vi "row1.vi"(2 "Array in":i32[](array[numeric])) -> (0 "Array out":i32[](array[numeric]), 1 "Enum":T1(ring))   [LabVIEW 2016]
uses:
  <vilib>/NXT/Block Support/NXT_OutputPort.ctl
  <vilib>/NXT/Block Support/NXT_InputPort.ctl
  <vilib>/NXT/Subs/ColorSensorColors.ctl
  <vilib>/NXT/NXTIO Xnodes/NXTIONodeSubVIs/NXTStopMotors.vi
  <vilib>/NXT/NXTIO Xnodes/NXTIONodeSubVIs/NXTMotorRunDistance.vi
  <vilib>/NXT/NXTIO Xnodes/NXTIONodeSubVIs/LEGOMotorStatus.vi
  <vilib>/NXT/NXTIO Xnodes/NXTIONodeSubVIs/NXTMoveMotors.vi
  <vilib>/NXT/NXTIO Xnodes/NXTIONodeSubVIs/LEGOResetMotors.vi
  <vilib>/NXT/Subs/LVHSConnector.ctl
  <vilib>/NXT/NXTIO Xnodes/AddressXNode/NXTIOAddress.xnode
  <vilib>/NXT/NXTIO Xnodes/NXTIOXNode/NXTIO.xnode
  <vilib>/NXT/LegoClasses/BrickReference/BrickReference.lvclass
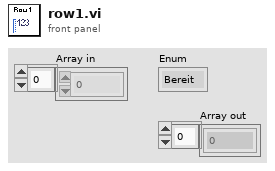
[diagram p1: front panel]
types:
  T1 = enum16{"Bereit", "Move 1", "Reference_pos", "Wait", "row1_check", "row2_check", "row3_check", "return", "move2", "move3", "move4", "move5", "end"}
  T2 = enum16{"forward", "pause1", "right1", "pause2", "right2", "pause3", "end"}
  T3 = typedef "NXT_OutputPort.ctl" = u8
  T4 = typedef "ColorSensorColors.ctl" = enum16{"No Color", "Black", "Blue", "Green", "Yellow", "Red", "White", "Brown"}
  T5 = cluster{"Output Port":T3, "Output Port 2":T3, "Output Port 3":T3}
  T6 = typedef "LVHSConnector.ctl" = refnum<class "BrickReference.lvclass">
  T7 = typedef "NXT_InputPort.ctl" = u32
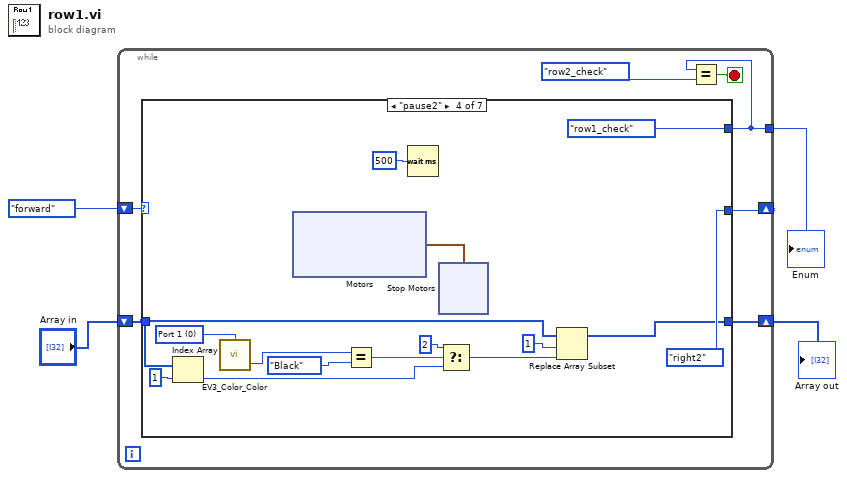
[diagram p0: block diagram]
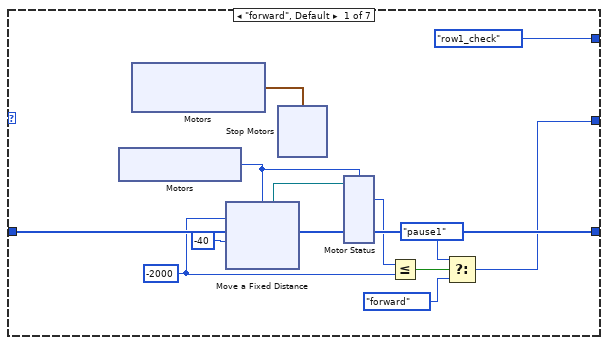
[diagram p2: hidden frame]
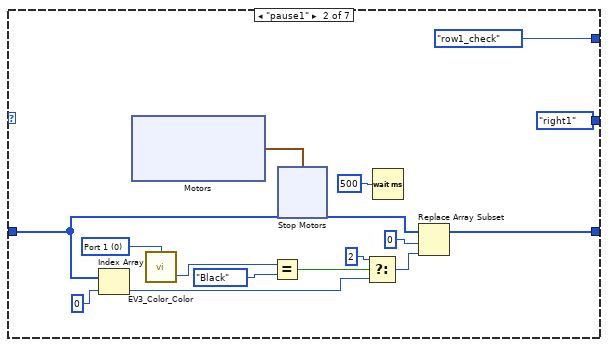
[diagram p3: hidden frame]
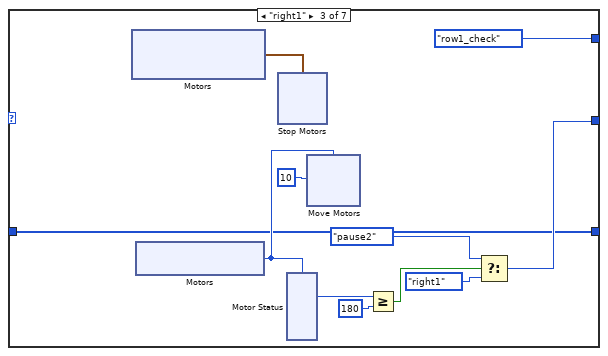
[diagram p4: hidden frame]
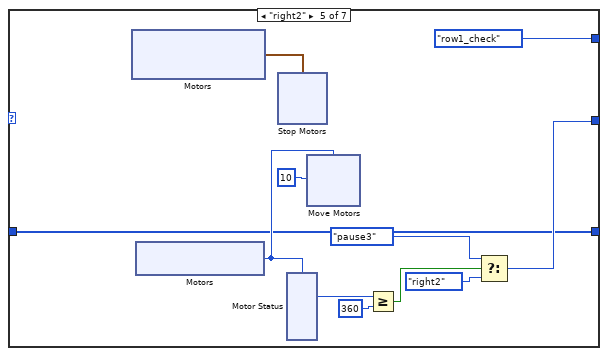
[diagram p5: hidden frame]
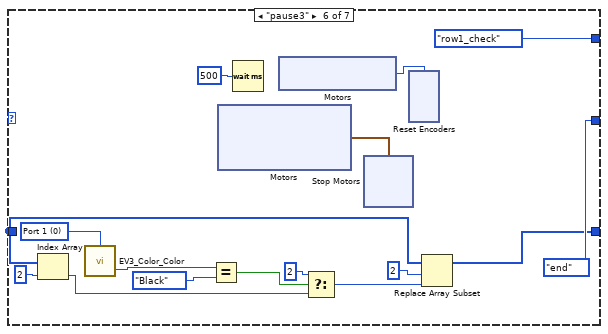
[diagram p6: hidden frame]
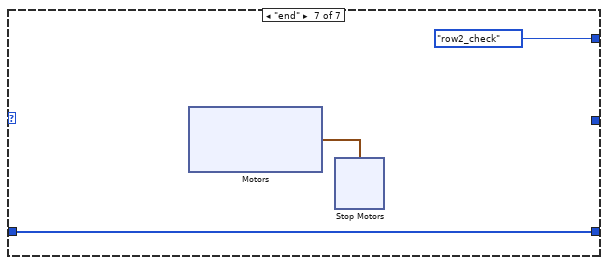
[diagram p7: hidden frame]
diagram:
  n1 = while {
    shift-right: [w10] -> _
    shift-left: T2."forward" -> [w11]
    tunnel: [w9] -> w2
    shift-right: [w7] -> w3
    shift-left: "Array in" -> [w8]
    stop <- w5 stop-if-true
    n2 = case shown="\"pause2\"" w11 {
      tunnel: [w15 T2."right1" w73 T2."right2" w129 T2."end" _] -> w10
      tunnel: [T1."row1_check" T1."row1_check" T1."row1_check" T1."row1_check" T1."row1_check" T1."row1_check" T1."row2_check"] -> w9
      tunnel: [w21 w49 w71 w105 w125 w158 w185] -> w7
      tunnel: w8 -> [w21 w51 w71 w106 w125 w159 w185]
      frame "forward", Default {
        w18 = -2000 ("Distance 1")
        n3 = xnode "Motors"() -> ("Motor"=w17:T3)
        n4 = xnode "Motors"() -> ("Motor"=w23:cluster{"Port":T3, "Port":T3})
        n5 = xnode "Move a Fixed Distance"("Speed 1"=i8 -40, "Distance 1"=w18, "Motors"=w17) -> ("NXT/EV3"=w16:T6)  [unwired: 1 in]
        n6 = xnode "Stop Motors"("Motors"=w23) -> ()  [unwired: 1 in, 1 out]
        n7 = xnode "Motor Status"("Motors"=w17, "NXT/EV3"=w16) -> ("Position 1"=w19:i32)  [unwired: 2 out]
        n8 = Less Or Equal?(x=w19, y=w18) -> (x <= y?=w12:bool)
        n9 = Select(t=T2."pause1", s=w12, f=T2."forward") -> (s? t:f=w15:T2)
      }
      frame "pause1" {
        w62 = T7 0 items=["Port 1", "Port 2", "Port 3", "Port 4"] ("Port (Port 1)")
        n10 = Index Array(array=w51, index=0 ("disabled index (col)")) -> (element=w50:i32)
        n11 = xnode "Motors"() -> ("Motor"=w63:cluster{"Port":T3, "Port":T3, "Port":T3})
        n12 = call <vilib>:"EV3_Color_Color.vi"("Port (Port 1)"=w62) -> ("Detected Color"=w61:T4)  [unwired: 2 in, 1 out]
        n13 = Equal?(x=w61, y=ColorSensorColors."Black") -> (x = y?=w58:bool)
        n14 = xnode "Stop Motors"("Motors"=w63) -> ()  [unwired: 1 in, 1 out]
        n15 = Select(t=2 ("disabled index (col)"), s=w58, f=w50) -> (s? t:f=w54:i32)
        n16 = Wait (ms)(milliseconds to wait=u32 500) -> ()  [unwired: 1 out]
        n17 = Replace Array Subset(array=w51, new element=w54, index=0 ("index (row)")) -> (w49:i32[])
      }
      frame "right1" {
        n18 = xnode "Motors"() -> ("Motor"=w78:cluster{"Port":T3, "Port":T3})
        n19 = xnode "Motors"() -> ("Motor"=w79:T3)
        n20 = xnode "Stop Motors"("Motors"=w78) -> ()  [unwired: 1 in, 1 out]
        n21 = xnode "Motor Status"("Motors"=w79) -> ("Position 1"=w77:i32)  [unwired: 1 in, 2 out]
        n22 = xnode "Move Motors"("Power/Speed 1"=i8 10, "Motors"=w79) -> ()  [unwired: 1 in, 1 out]
        n23 = Greater Or Equal?(x=w77, y=180) -> (x >= y?=w75:bool)
        n24 = Select(t=T2."pause2", s=w75, f=T2."right1") -> (s? t:f=w73:T2)
      }
      frame "pause2" {
        w116 = T7 0 items=["Port 1", "Port 2", "Port 3", "Port 4"] ("Port (Port 1)")
        n25 = Index Array(array=w106, index=1 ("disabled index (col)")) -> (element=w107:i32)
        n26 = call <vilib>:"EV3_Color_Color.vi"("Port (Port 1)"=w116) -> ("Detected Color"=w115:T4)  [unwired: 2 in, 1 out]
        n27 = xnode "Motors"() -> ("Motor"=w117:cluster{"Port":T3, "Port":T3, "Port":T3})
        n28 = Equal?(x=w115, y=ColorSensorColors."Black") -> (x = y?=w112:bool)
        n29 = Wait (ms)(milliseconds to wait=u32 500) -> ()  [unwired: 1 out]
        n30 = xnode "Stop Motors"("Motors"=w117) -> ()  [unwired: 1 in, 1 out]
        n31 = Select(t=2 ("disabled index (col)"), s=w112, f=w107) -> (s? t:f=w103:i32)
        n32 = Replace Array Subset(array=w106, new element=w103, index=1 ("disabled index (col)")) -> (w105:i32[])
      }
      frame "right2" {
        n33 = xnode "Motors"() -> ("Motor"=w132:cluster{"Port":T3, "Port":T3})
        n34 = xnode "Motors"() -> ("Motor"=w133:T3)
        n35 = xnode "Stop Motors"("Motors"=w132) -> ()  [unwired: 1 in, 1 out]
        n36 = xnode "Motor Status"("Motors"=w133) -> ("Position 1"=w128:i32)  [unwired: 1 in, 2 out]
        n37 = xnode "Move Motors"("Power/Speed 1"=i8 10, "Motors"=w133) -> ()  [unwired: 1 in, 1 out]
        n38 = Greater Or Equal?(x=w128, y=360) -> (x >= y?=w131:bool)
        n39 = Select(t=T2."pause3", s=w131, f=T2."right2") -> (s? t:f=w129:T2)
      }
      frame "pause3" {
        w171 = T7 0 items=["Port 1", "Port 2", "Port 3", "Port 4"] ("Port (Port 1)")
        n40 = Index Array(array=w159, index=2 ("disabled index (col)")) -> (element=w162:i32)
        n41 = call <vilib>:"EV3_Color_Color.vi"("Port (Port 1)"=w171) -> ("Detected Color"=w170:T4)  [unwired: 2 in, 1 out]
        n42 = Equal?(x=w170, y=ColorSensorColors."Black") -> (x = y?=w167:bool)
        n43 = xnode "Motors"() -> ("Motor"=w172:cluster{"Port":T3, "Port":T3, "Port":T3})
        n44 = Wait (ms)(milliseconds to wait=u32 500) -> ()  [unwired: 1 out]
        n45 = xnode "Motors"() -> ("Motor"=w157:T3)
        n46 = Select(t=2 ("disabled index (col)"), s=w167, f=w162) -> (s? t:f=w160:i32)
        n47 = xnode "Stop Motors"("Motors"=w172) -> ()  [unwired: 1 in, 1 out]
        n48 = xnode "Reset Encoders"("Motors"=w157) -> ()  [unwired: 1 in, 1 out]
        n49 = Replace Array Subset(array=w159, new element=w160, index=2 ("disabled index (col)")) -> (w158:i32[])
      }
      frame "end" {
        n50 = xnode "Motors"() -> ("Motor"=w186:cluster{"Port":T3, "Port":T3, "Port":T3})
        n51 = xnode "Stop Motors"("Motors"=w186) -> ()  [unwired: 1 in, 1 out]
      }
    }
    n52 = Equal?(x=w9, y=T1."row2_check") -> (x = y?=w5:bool)
  }
  "Array out" <- w3
  "Enum" <- w2
